vi "Write Flow Control Valve Compensator.vi"(10 "Flow Control Valve Compensator":T1={"PID Gains"={"Proportional Gain (Kc)"=1.0, "Integral Time (Ti, min)"=0.01, "Derivative Time (Td, min)"=0.0}, "Flow Control Valve Output Range"={"High"=0.0, "Low"=0.0}} {"Flow Control Valve Output Range"."Low" min=-888.0 max=888.0 format="%.2f"; "Flow Control Valve Output Range"."High" min=-888.0 max=888.0 format="%.2f"; "PID Gains"."Derivative Time (Td, min)" format="%.3f"; "PID Gains"."Integral Time (Ti, min)" format="%.3f"; "PID Gains"."Proportional Gain (Kc)" format="%.3f"}, 11 "FlowControlValveCompensator in":refnum<class "FlowControlValveCompensator.lvclass">) -> (3 "FlowControlValveCompensator out":refnum<class "FlowControlValveCompensator.lvclass">)   [LabVIEW 2013, in "FlowControlValveCompensator.lvclass"]
uses:
  FlowControlValveCompensator.lvclass
  Configuration/FlowControlValveCompensator.ctl
  Configuration/PIDGains.ctl
  Configuration/FlowControlValveOutputRange.ctl
  FlowControlValveCompensator.lvclass/FlowControlValveCompensator.ctl
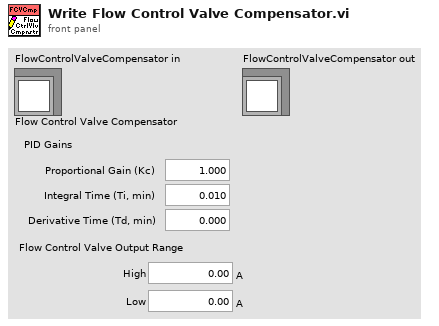
[diagram p1: front panel]
types:
  T1 = typedef "FlowControlValveCompensator.ctl" = cluster{"PID Gains":T2, "Flow Control Valve Output Range":T3}
  T2 = typedef "PIDGains.ctl" = cluster{"Proportional Gain (Kc)":dbl, "Integral Time (Ti, min)":dbl, "Derivative Time (Td, min)":dbl}
  T3 = typedef "FlowControlValveOutputRange.ctl" = cluster{"High":dbl[unit], "Low":dbl[unit]}
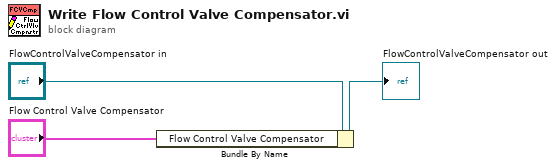
[diagram p0: block diagram]
diagram:
  n1 = Bundle By Name(cluster="FlowControlValveCompensator in", "Flow Control Valve Compensator"="Flow Control Valve Compensator") -> (→"FlowControlValveCompensator out":refnum<class "FlowControlValveCompensator.lvclass">)
